vi "Parse-attribute.vi"(8 "error in (no error)":errorcluster, 10 "String in":string, 11 "XYCalFactor in":refnum<class "XYCalFactor.lvclass">) -> (0 "error out":errorcluster, 1 "Valid attribute?":bool, 2 "Remaining string":string, 3 "XYCalFactor out":refnum<class "XYCalFactor.lvclass">)   [LabVIEW 2013, in "HardwareCharacterization.lvlib" / "XYCalFactor.lvclass"]
uses:
  XYCalFactor.lvclass
  Attributes.ctl
  Attribute-ID.ctl
  Attribute-XML.lvclass/Attribute-XML.ctl
  ID.lvclass/ID.ctl
  XYCalFactor.lvclass/XYCalFactor.ctl
  Write Attribute.vi
  Write ID-attribute.vi
  Write XY unit scale factor.vi
  Attribute-XML.lvclass
  ID.lvclass
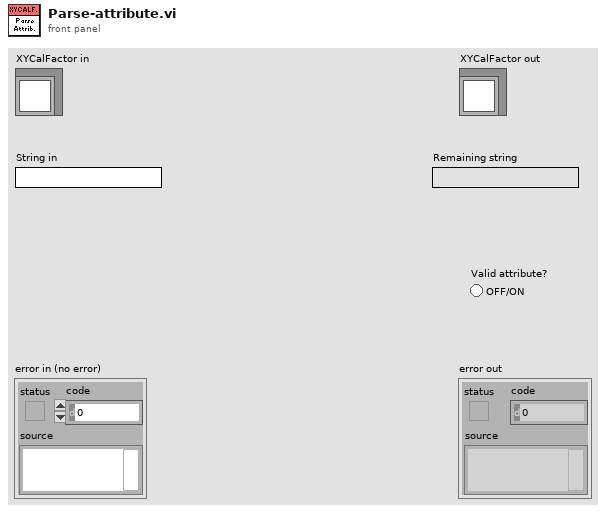
[diagram p1: front panel]
types:
  T1 = typedef "HardwareCharacterization.lvlib/ID.lvclass/Attribute-ID.ctl" = enum16{"FieldOffset", "TransformEnable", "Transform", "Units", "XYCalFactor", "EnableLaser", "JumpDelay", "MarkDelay", "PolyDelay", "LaserOnDelay", "LaserOffDelay", "JumpSpeed", "MarkSpeed", "LaserPowerDelay", "LaserEnableDelay", "LaserPower", "Offset"}
  T2 = typedef "HardwareCharacterization.lvlib/Attribute-XML.lvclass/Attributes.ctl" = enum16{"id"}
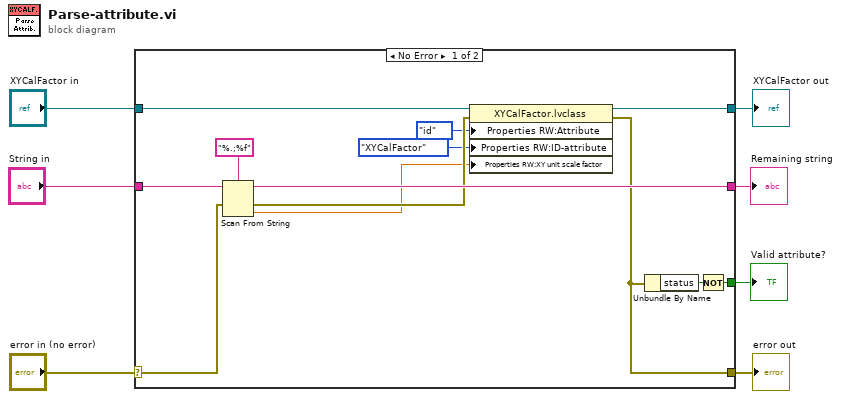
[diagram p0: block diagram]
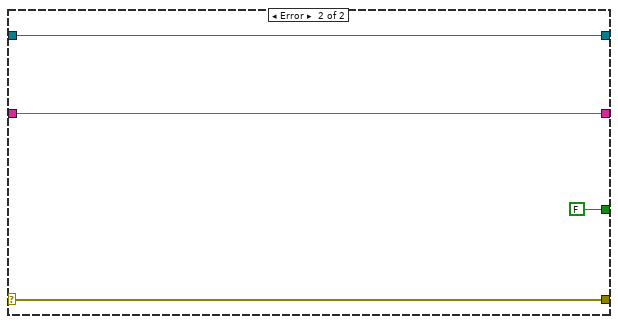
[diagram p2: hidden frame]
diagram:
  n1 = case shown="No Error" "error in (no error)" {
    selector: "error in (no error)" -> [w17 w24]
    tunnel: [w13 w24] -> w6
    tunnel: [w14 w23] -> w4
    tunnel: "XYCalFactor in" -> [w11 w23]
    tunnel: "String in" -> [w18 w22]
    tunnel: [w16 FALSE] -> w2
    tunnel: [w15 w22] -> w1
    frame No Error {
      n2 = Scan From String(format string="%.;%f", input string=w18, error in=w17) -> (remaining string=w15:string, error out=w12:errorcluster, output 1=w8:dbl)  [unwired: 2 in, 1 out]
      n3 = property class="XYCalFactor.lvclass"(reference=w11, error in=w12, "Properties RW:Attribute"=Attributes."id" ("Attribute"), "Properties RW:ID-attribute"=Attribute-ID."XYCalFactor" ("ID-attribute"), "Properties RW:XY unit scale factor"=w8) -> (reference out=w14:refnum<class "XYCalFactor.lvclass">, error out=w13:errorcluster)
      n4 = Unbundle By Name(w13) -> ("status"=w19:bool)
      n5 = Not(x=w19) -> (.not. x?=w16:bool)
    }
    frame Error {
    }
  }
  "error out" <- w6
  "XYCalFactor out" <- w4
  "Remaining string" <- w1
  "Valid attribute?" <- w2
